vi "Balance_change.vi"(8 "error in (no error)":errorcluster, 9 "Amount":dbl, 10 "Depost/Withdraw":bool, 11 "Database_handler in":refnum<class "Database_handler.lvclass">) -> (0 "error out":errorcluster, 3 "Database_handler out":refnum<class "Database_handler.lvclass">)   [LabVIEW 2025, in "Database_handler.lvlib" / "Database_handler.lvclass"]
uses:
  Database_handler.lvclass
  Database_handler.lvclass/Database_handler.ctl
  DB_fb_tocont Messages/Balance_fb Msg/Balance_fb Msg.lvclass/Balance_fb Msg.ctl
  <vilib>/ActorFramework/Message Enqueuer/Message Enqueuer.lvclass/Message Enqueuer.ctl
  <vilib>/ActorFramework/Message Enqueuer/Enqueue.vi
  DB_fb_tocont Messages/Balance_fb Msg/Balance_fb Msg.lvclass
  <vilib>/ActorFramework/Message Priority Queue/Priority Enqueue.vi
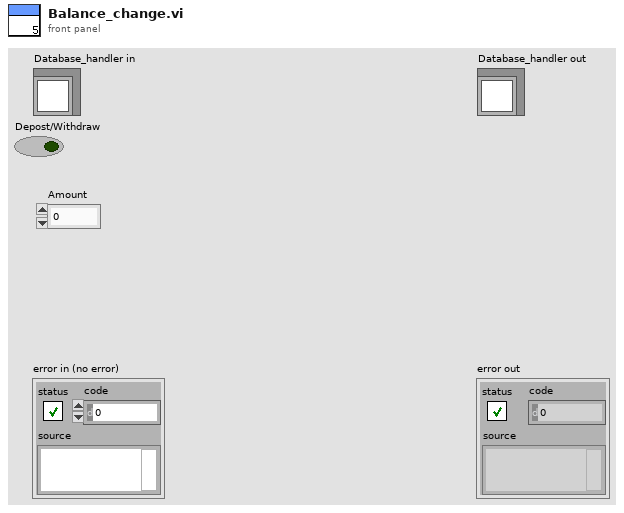
[diagram p1: front panel]
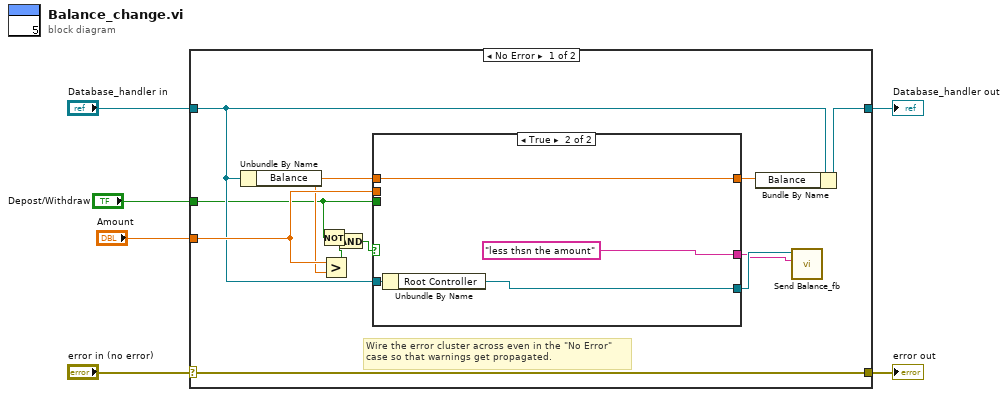
[diagram p0: block diagram]
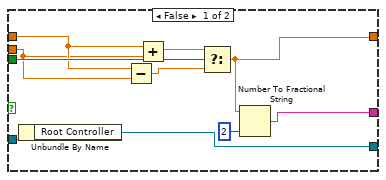
[diagram p2: hidden frame]
diagram:
  n1 = case shown="No Error" "error in (no error)" {
    selector: "error in (no error)" -> [w18 w34]
    tunnel: [w18 w34] -> w5
    tunnel: [w15 w33] -> w3
    tunnel: "Database_handler in" -> [w13 w33]
    tunnel: "Depost/Withdraw" -> [w8 _]
    tunnel: "Amount" -> [w17 _]
    frame No Error {
      # "Wire the error cluster across even in the \"No Error\"\ncase so that warnings get propagated."
      n2 = Unbundle By Name(w13) -> ("Balance"=w16:dbl)
      n3 = Not(x=w8) -> (.not. x?=w7:bool)
      n4 = Greater?(x=w17, y=w16) -> (0:w9:bool)
      n5 = And(x=w7, y=w9) -> (x .and. y?=w10:bool)
      n6 = case shown="True" w10 {
        tunnel: w8 -> [w28 _]
        tunnel: w16 -> [w27 w32]
        tunnel: w17 -> [w24 _]
        tunnel: [w23 w32] -> w14
        tunnel: w13 -> [w20 w30]
        tunnel: [w21 "less thsn the amount"] -> w11
        tunnel: [w19 w29] -> w12
        frame False {
          n7 = Unbundle By Name(w20) -> ("Root Controller"=w19:refnum<class "Message Enqueuer.lvclass">)
          n8 = Subtract(x=w27, y=w24) -> (x-y=w25:dbl)
          n9 = Add(x=w27, y=w24) -> (x+y=w26:dbl)
          n10 = Select(t=w26, s=w28, f=w25) -> (s? t:f=w23:dbl)
          n11 = Number To Fractional String(number=w23, precision (6)=i16 2) -> (F-format string=w21:string)  [unwired: 2 in]
        }
        frame True {
          n12 = Unbundle By Name(w30) -> ("Root Controller"=w29:refnum<class "Message Enqueuer.lvclass">)
        }
      }
      n13 = Bundle By Name(cluster=w13, "Balance"=w14) -> (w15:refnum<class "Database_handler.lvclass">)
      n14 = call "Send Balance_fb.vi"("Balance"=w11, "Message Enqueuer"=w12) -> ()  [unwired: 8 in, 2 out]
    }
    frame Error {
    }
  }
  "error out" <- w5
  "Database_handler out" <- w3
